vi "Cut from start.vi"(2 "bytes to cut":i32=-1, 3 "bytestream in":refnum<class "Bytestream.lvclass">) -> (0 "data":u8[](array[numeric]) format="%02x", 1 "bytestream out":refnum<class "Bytestream.lvclass">)   [LabVIEW 2020, in "NI_Bytestream.lvlib" / "Bytestream.lvclass"]
uses:
  <vilib>/Array/Bytestream/Bytestream.lvclass
  <vilib>/Array/Bytestream/Bytestream.lvclass/Bytestream.ctl
  <vilib>/Array/Bytestream/Get Logical Datum.vi
  <vilib>/Array/Bytestream/Count Datums.vi
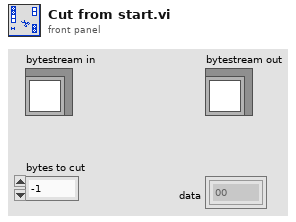
[diagram p1: front panel]
types:
  T1 = typedef "NI_Bytestream.lvlib/Bytestream.lvclass/Datum.ctl" = cluster{"array":u8[], "index":i32}
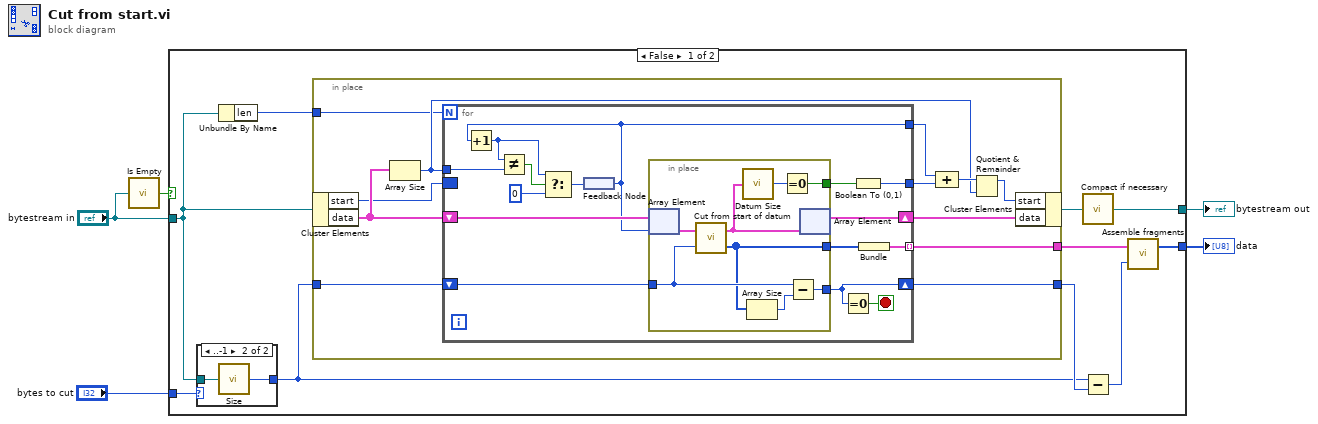
[diagram p0: block diagram]
diagram:
  n1 = call <vilib>:"Is Empty.vi"("a"="bytestream in") -> ("empty?"=w1:bool)
  n2 = case shown="False" w1 {
    tunnel: [w12 _] -> w5
    tunnel: [w10 w54] -> w4
    tunnel: "bytestream in" -> [w9 w54]
    tunnel: "bytes to cut" -> [w8 _]
    frame False {
      n3 = case shown="..-1" w8 {
        selector: w8 -> [w51 _]
        tunnel: w9 -> [_ w53]
        tunnel: [w51 w52] -> w7
        frame Default {
        }
        frame ..-1 {
          n4 = call <vilib>:"Size.vi"("ByteArrayTuple in"=w53) -> ("size"=w52:i32)
        }
      }
      n5 = Unbundle By Name(w9) -> ("len"=w6:i32)
      n6 = in-place {
        in-place-border: w7 -> [w27]
        in-place-border: [w25] -> w15
        in-place-border: [w24] -> w14
        in-place-border: w6 -> [w18]
        n7 = in-place-cluster #1(w9) -> ("start"=w17:i32, "data"=w26:T1[])
        n8 = Array Size(array=w26) -> (size(s)=w19:i32)
        n9 = for {
          N: w18 -> [_]
          shift-right: [w39] -> w25
          shift-left: w27 -> [w42]
          shift-right: [w41] -> w23
          shift-left: w26 -> [w36]
          tunnel: [w37] -> w24 mode=indexing
          tunnel: [w32] -> w22
          tunnel: [w34] -> w20
          tunnel: w19 -> [w31]
          border: w17 -> [_]
          stop <- w40 stop-if-true
          n10 = feedback #2() -> (w32:i32)
          n11 = Increment(x=w32) -> (x+1=w29:i32)
          n12 = Not Equal?(x=w29, y=w31) -> (x != y?=w33:bool)
          n13 = Select(t=w29, s=w33, f=0 ("t")) -> (s? t:f=w30:i32)
          n14 = feedback-in #2(w30) -> ()
          n15 = in-place {
            in-place-border: w42 -> [w49]
            in-place-border: [w48] -> w39
            in-place-border: [w46] -> w38
            in-place-border: [w43] -> w35
            n16 = in-place-array #3(w36, w32) -> (w47:T1)
            n17 = call <vilib>:"Cut from start of datum.vi"("length"=w49, "datum"=w47) -> ("data"=w46:u8[], "datum out"=w45:T1)
            n18 = call <vilib>:"Datum Size.vi"("datum"=w45) -> ("size"=w44:i32)
            n19 = Array Size(array=w46) -> (size(s)=w50:i32)
            n20 = Equal To 0?(x=w44) -> (x = 0?=w43:bool)
            n21 = Subtract(x=w49, y=w50) -> (x-y=w48:i32)
            n22 = in-place-array #3(w45) -> (w41:T1[])  [unwired: 1 out]
          }
          n23 = Equal To 0?(x=w39) -> (x = 0?=w40:bool)
          n24 = Boolean To (0,1)(Boolean=w35) -> (0, 1=w34:i16)
          n25 = Bundle("data"=w38) -> (w37:cluster{"data":u8[]})  [unwired: 1 in]
        }
        n26 = Compound Arithmetic op=ADD(w22, w20) -> (w21:i32)
        n27 = Quotient & Remainder(x=w21, y=w19) -> (x-y*floor(x/y)=w16:i32)  [unwired: 1 out]
        n28 = in-place-cluster #1("start"=w16, "data"=w23) -> (w11:refnum<class "Bytestream.lvclass">)
      }
      n29 = call <vilib>:"Compact if necessary.vi"("bytestream"=w11) -> ("bytestream out"=w10:refnum<class "Bytestream.lvclass">)
      n30 = Subtract(x=w7, y=w15) -> (x-y=w13:i32)
      n31 = call <vilib>:"Assemble fragments.vi"("Numeric"=w13, "Array in"=w14) -> ("Array out"=w12:u8[])  [unwired: 1 in]
    }
    frame True {
    }
  }
  "bytestream out" <- w4
  "data" <- w5
